vi "VisitSites.vi"(0 "Microsites":T3(array[cluster]), 4 "Path":path, 7 "UiDefinition":T2, 13 "CurrentPositionIndex":i32) -> ()   [LabVIEW 2020]
uses:
  UIReferences.ctl
  C:/Users/User/Desktop/Automation/CurrentVersion/LabviewDXFViewer/bin/Release/LabviewDXFViewer.exe
  LabviewDXFViewer/bin/Release/LabviewDXFViewer.exe
  Control 2.ctl
  <vilib>/Utility/file.llb/Write Delimited Spreadsheet (string).vi
panel:
  out "error out 17":errorcluster
  out "error out 16":errorcluster
  out "error out 15":errorcluster
  out "error out 14":errorcluster
  out "error out 13":errorcluster
  out "error out 12":errorcluster
  out "error out 11":errorcluster
  out "error out 10":errorcluster
  out "error out 9":errorcluster
  out "error out 8":errorcluster
  out "error out 7":errorcluster
  out "error out 6":errorcluster
  out "error out 5":errorcluster
  out "error out 4":errorcluster
  out "IV Curves":T1
  out "error out 3":errorcluster
  out "error out 2":errorcluster
  out "error out":errorcluster
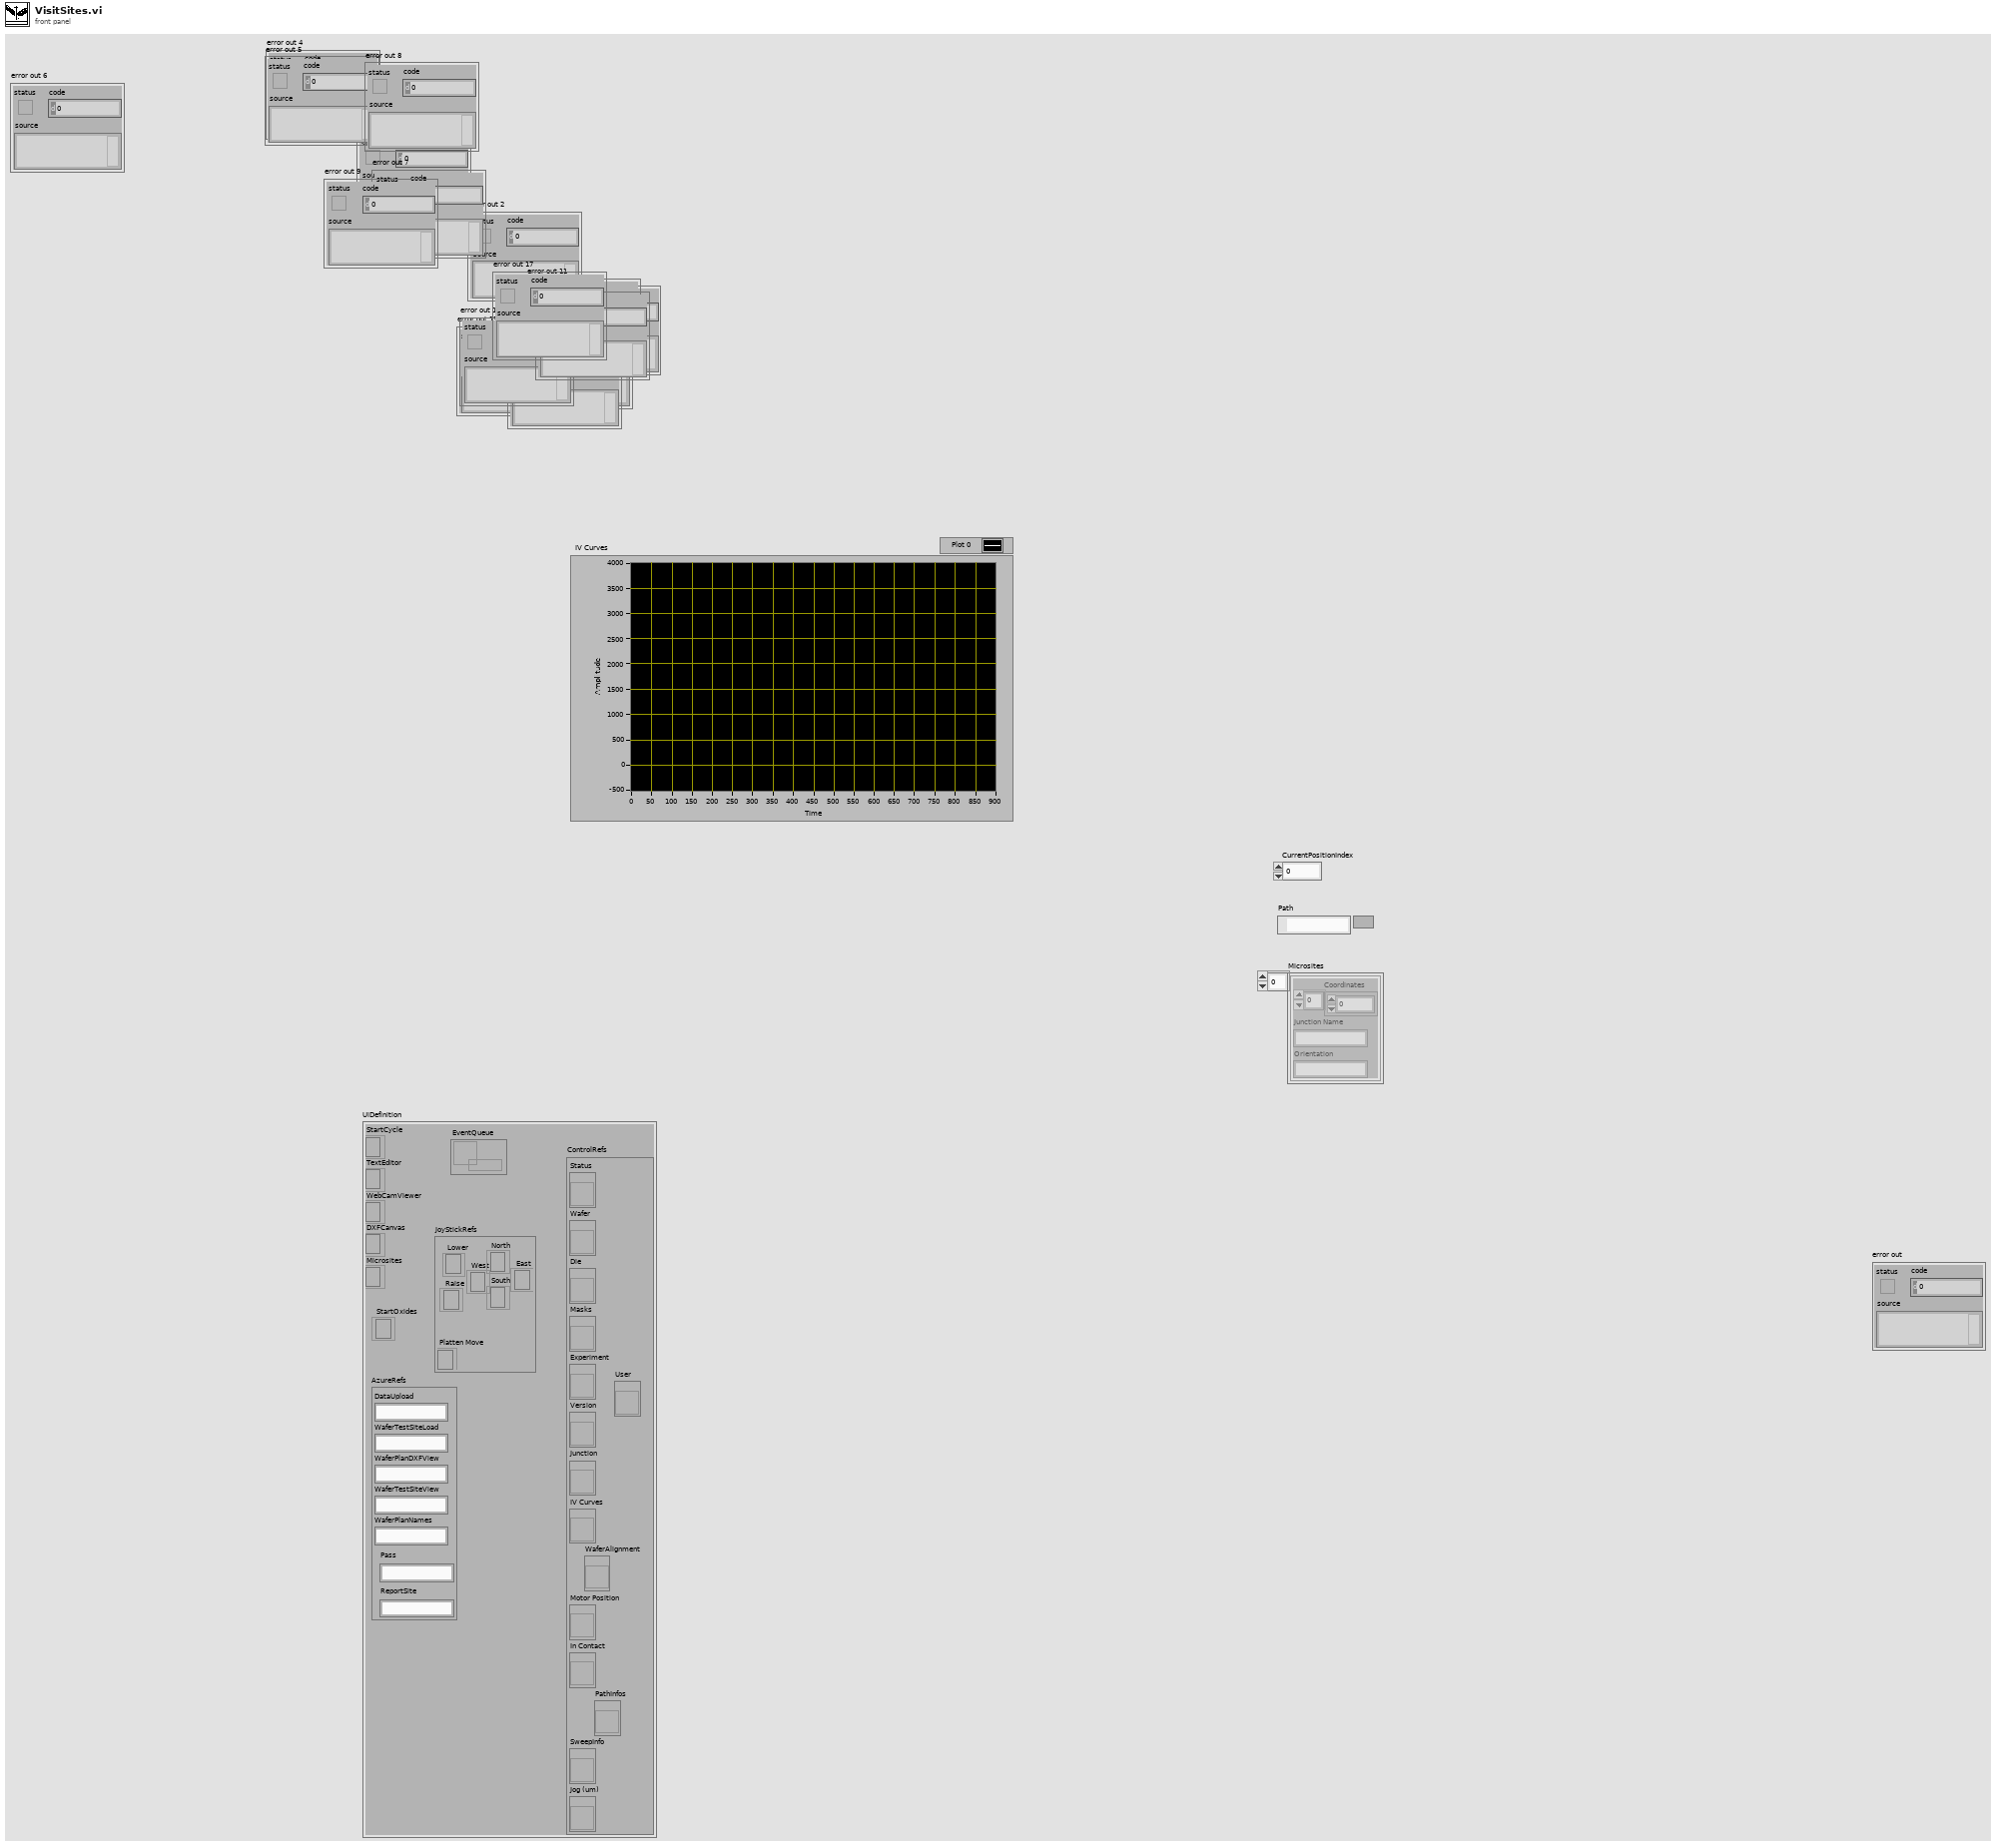
[diagram p1: front panel]
types:
  T1 = typedef "Control 2.ctl" = cluster{"Y":dbl[], "Current (A)":dbl[]}
  T2 = typedef "UIReferences.ctl" = cluster{"StartCycle":refnum<k24>, "TextEditor":refnum<k24>, "WebCamViewer":refnum<k24>, "DXFCanvas":refnum<k24>, "Microsites":refnum<k24>, "JoyStickRefs":cluster{"North":refnum<k24>, "Lower":refnum<k24>, "Raise":refnum<k24>, "Platten Move":refnum<k24>, "West":refnum<k24>, "East":refnum<k24>, "South":refnum<k24>}, "AzureRefs":cluster{"DataUpload":string, "WaferTestSiteLoad":string, "WaferPlanDXFView":string, "WaferTestSiteView":string, "WaferPlanNames":string, "Pass":string, "ReportSite":string}, "ControlRefs":cluster{"Status":refnum<vi>, "Wafer":refnum<vi>, "Die":refnum<vi>, "Masks":refnum<vi>, "Experiment":refnum<vi>, "Version":refnum<vi>, "Junction":refnum<vi>, "IV Curves":refnum<vi>, "Motor Position":refnum<vi>, "In Contact":refnum<vi>, "SweepInfo":refnum<vi>, "Jog (um)":refnum<vi>, "PathInfos":refnum<vi>, "User":refnum<vi>, "WaferAlignment":refnum<vi>}, "EventQueue":refnum<queue>, "StartOxides":refnum<k24>}
  T3 = cluster{"Coordinates":dbl[], "Junction Name":string, "Orientation":string}[]
  T4 = cluster{"Coordinates":dbl[], "Junction Name":string, "Orientation":string}
  T5 = typedef "WaferAlignmentType.ctl" = cluster{"Wafer Units to microns":dbl, "Rotation Misalign":dbl[], "Scale Misalign":dbl, "Steps Per micron":dbl, "Position 1":i32[], "Position 2":i32[], "Lift Distance":i32, "Position 3":i32[], "Jog Height":i32}
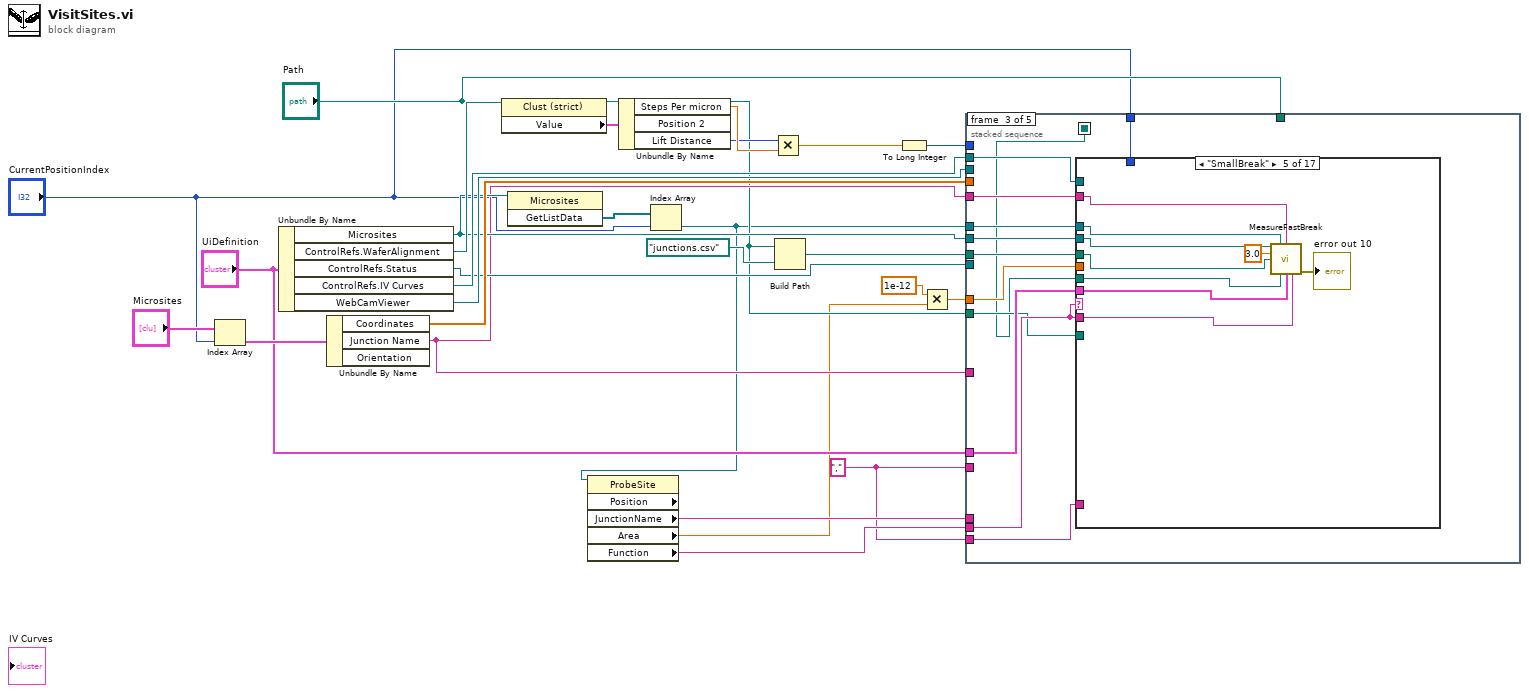
[diagram p0: block diagram]
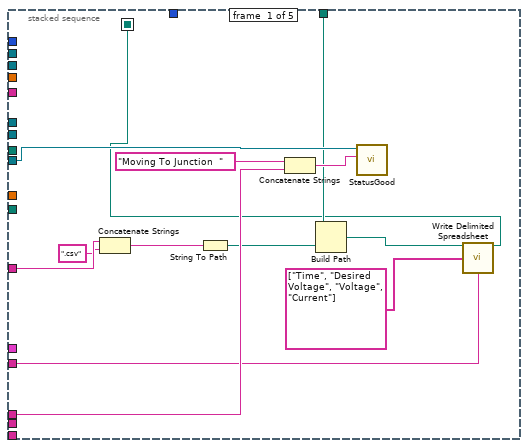
[diagram p2: hidden frame]
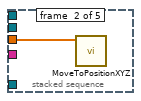
[diagram p3: hidden frame]
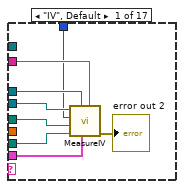
[diagram p4: hidden frame]
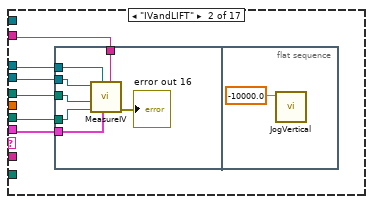
[diagram p5: hidden frame]
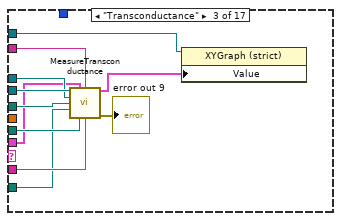
[diagram p6: hidden frame]
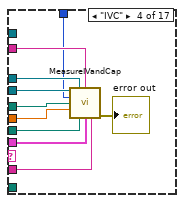
[diagram p7: hidden frame]
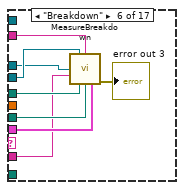
[diagram p8: hidden frame]
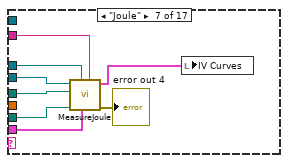
[diagram p9: hidden frame]
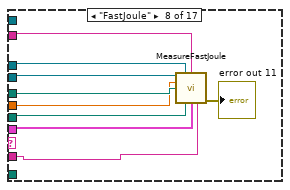
[diagram p10: hidden frame]
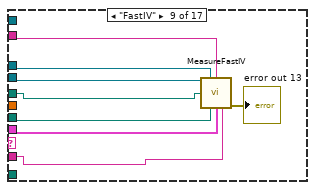
[diagram p11: hidden frame]
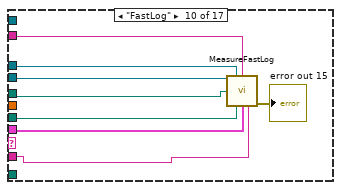
[diagram p12: hidden frame]
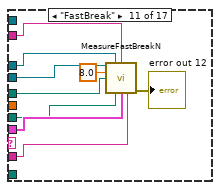
[diagram p13: hidden frame]
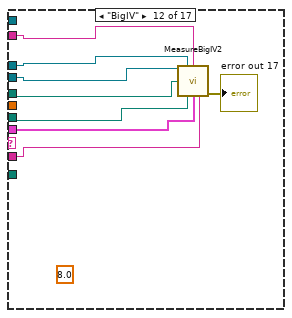
[diagram p14: hidden frame]
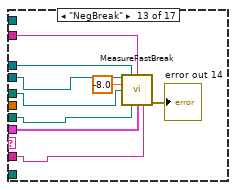
[diagram p15: hidden frame]
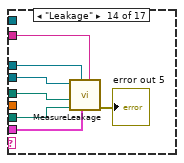
[diagram p16: hidden frame]
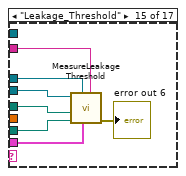
[diagram p17: hidden frame]
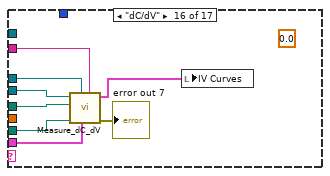
[diagram p18: hidden frame]
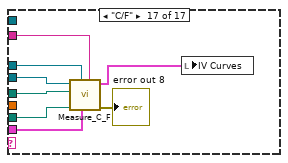
[diagram p19: hidden frame]
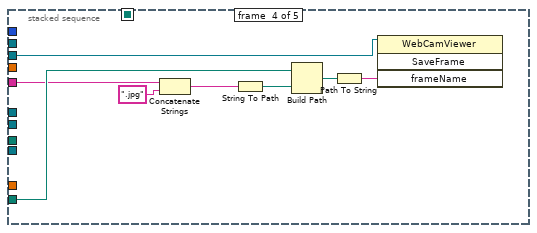
[diagram p20: hidden frame]
diagram:
  w6 = "," ("delimiter (\\t)")
  n1 = Index Array(array="Microsites", index="CurrentPositionIndex") -> (element=w22:T4)
  n2 = Unbundle By Name("UiDefinition") -> ("Microsites"=w9:refnum<k24>, "ControlRefs.WaferAlignment"=w20:refnum<vi>, "ControlRefs.Status"=w7:refnum<vi>, "ControlRefs.IV Curves"=w15:refnum<vi>, "WebCamViewer"=w13:refnum<k24>)
  n3 = Unbundle By Name(w22) -> ("Coordinates"=w25:dbl[], "Junction Name"=w5:string)  [unwired: 1 out]
  n4 = property class="Clust (strict)"(reference=w20) -> ("Value"=w19:T5)  [unwired: 1 in, 2 out]
  n5 = invoke class="Microsites" method="GetListData"(reference=w9) -> ("GetListData"=w21:refnum<k24>[])  [unwired: 2 in, 2 out]
  n6 = Unbundle By Name(w19) -> ("Steps Per micron"=w17:dbl, "Lift Distance"=w16:i32)  [unwired: 1 out]
  n7 = Index Array(array=w21, index="CurrentPositionIndex") -> (element=w2:refnum<k24>)
  n8 = property class="ProbeSite" props=["Position", "JunctionName", "Area", "Function"](reference=w2) -> ("JunctionName"=w8:string, "Area"=w3:dbl, "Function"=w10:string)  [unwired: 1 in, 3 out]
  n9 = Multiply(x=w16, y=w17) -> (x*y=w18:dbl)
  n10 = Build Path(base path="Path", name or relative path=path "junctions.csv") -> (appended path=w26:path)
  n11 = To Long Integer(number=w18) -> (32bit integer=w27:i32)
  n12 = Multiply(x=1e-12, y=w3) -> (x*y=w12:dbl)
  n13 = stacked-sequence {
    seq-local: [w28 _ _ _ _] -> [_ _ w43 _ _]
    tunnel: w27 -> [_ _ _ _ w212]
    tunnel: w26 -> [_ _ w53 _ _]
    tunnel: w25 -> [_ w41 _ _ _]
    tunnel: w5 -> [_ _ w52 w205 _]
    tunnel: w15 -> [_ _ w45 _ _]
    tunnel: "UiDefinition" -> [_ _ w50 _ _]
    tunnel: w6 -> [_ _ w51 _ _]
    tunnel: w13 -> [_ _ _ w210 _]
    tunnel: "Path" -> [_ _ w44 w209 _]
    tunnel: w12 -> [_ _ w49 _ _]
    tunnel: w10 -> [_ _ w46 _ _]
    tunnel: w9 -> [_ _ w48 _ _]
    tunnel: w2 -> [_ _ w47 _ _]
    tunnel: w8 -> [w38 _ _ _ _]
    tunnel: w7 -> [w37 _ _ _ _]
    tunnel: w6 -> [w32 _ _ _ _]
    tunnel: w5 -> [w31 _ _ _ _]
    tunnel: "Path" -> [w29 _ _ _ _]
    tunnel: "CurrentPositionIndex" -> [_ _ w42 _ _]
    frame #0 {
      n14 = Concatenate Strings(w31, ".csv" ("string")) -> (w34:string)
      n15 = String To Path(string=w34) -> (path=w35:path)
      n16 = Concatenate Strings("Moving To Junction  " ("Text.Text"), w38) -> (w40:string)
      n17 = Build Path(base path=w29, name or relative path=w35) -> (appended path=w36:path)
      n18 = call "StatusGood.vi"("Text.Text"=w40, "String in"=w37) -> ()  [unwired: 10 in]
      n19 = call-poly <vilib>:"Write Delimited Spreadsheet.vi"("file path (dialog if empty)"=w36, "1D data"=string[] ["Time", "Desired Voltage", "Voltage", "Current"], "delimiter (\\t)"=w32) -> ("new file path (Not A Path if cancelled)"=w28:path)  [unwired: 11 in, 1 out]
    }
    frame #1 {
      n20 = call "MoveToPositionXYZ.vi"("Array"=w41) -> ()  [unwired: 11 in]
    }
    frame #2 {
      n21 = case shown="\"SmallBreak\"" w46 {
        tunnel: w53 -> [w59 w64 w82 w96 w97 w113 w116 w124 w134 w142 w147 w159 w165 w176 w182 w191 w199]
        tunnel: w52 -> [w58 w67 w76 w95 w104 w107 w117 w129 w137 w145 w154 w158 w170 w175 w183 w190 w198]
        tunnel: w43 -> [w60 w63 w83 w94 w99 w112 w118 w123 w133 w141 w149 w160 w164 w174 w181 w189 w196]
        tunnel: w51 -> [_ _ _ _ _ _ _ _ _ _ _ _ _ _ _ _ _]
        tunnel: w50 -> [w57 w62 w80 w93 w100 w109 w115 w125 w132 w140 w150 w161 w167 w173 w180 w188 w197]
        tunnel: w49 -> [_ _ _ w92 _ _ _ w122 _ _ _ _ _ _ _ _ _]
        tunnel: w48 -> [w56 w65 w85 w91 w102 w111 w120 w127 w135 w143 w152 w156 w166 w177 w184 w192 w200]
        tunnel: w47 -> [w55 w66 w84 w90 w103 w110 w119 w128 w136 w144 w153 w157 w169 w178 w185 w193 w201]
        tunnel: w46 -> [_ _ w81 w89 w101 w108 _ w126 w131 w139 w151 w162 w168 _ _ _ _]
        tunnel: w45 -> [_ _ w79 _ _ _ _ _ _ _ _ _ _ _ _ _ _]
        tunnel: w44 -> [_ _ w77 _ _ _ _ _ _ _ _ _ _ _ _ _ _]
        tunnel: w42 -> [w54 _ _ w87 _ _ _ _ _ _ _ _ _ _ _ _ _]
        frame "IV", Default {
          n22 = call "MeasureIV.vi"("Junction Name"=w58, "UiDefinition"=w57, ".NET Refnum"=w55, "new file path (Not A Path if cancelled)"=w60, "appended path"=w59, "CurrentPositionIndex"=w54, ".NET Refnum in"=w56) -> ("error out"=→"error out 2":errorcluster)  [unwired: 4 in]
        }
        frame "IVandLIFT" {
          n23 = flat-sequence {
            tunnel: w67 -> [w73]
            tunnel: w66 -> [w72]
            tunnel: w65 -> [w71]
            tunnel: w64 -> [w70]
            tunnel: w63 -> [w69]
            tunnel: w62 -> [w68]
            frame #0 {
              n24 = call "MeasureIV.vi"("Junction Name"=w73, "UiDefinition"=w68, ".NET Refnum"=w72, "new file path (Not A Path if cancelled)"=w69, "appended path"=w70, ".NET Refnum in"=w71) -> ("error out"=→"error out 16":errorcluster)  [unwired: 5 in]
            }
            frame #1 {
              n25 = call "JogVertical.vi"("Numeric"=-10000.0) -> ()  [unwired: 11 in]
            }
          }
        }
        frame "Transconductance" {
          n26 = call "MeasureTransconductance.vi"(".NET Refnum in"=w85, "UiDefinition"=w80, "Junction Name"=w76, ".NET Refnum"=w84, "appended path"=w82, "Path"=w77, "new file path (Not A Path if cancelled)"=w83, "Function"=w81) -> ("Cluster"=w78:cluster{dbl[], dbl[]}, "error out"=→"error out 9":errorcluster)  [unwired: 6 in]
          n27 = property class="XYGraph (strict)"(reference=w79, "Value"=w78) -> ()  [unwired: 1 in, 2 out]
        }
        frame "IVC" {
          n28 = call "MeasureIVandCap.vi"(".NET Refnum in"=w91, ".NET Refnum"=w90, "Junction Name"=w95, "CurrentPositionIndex"=w87, "appended path"=w96, "Numeric"=w92, "new file path (Not A Path if cancelled)"=w94, "UiDefinition"=w93, "Function"=w89) -> ("error out"=→"error out":errorcluster)  [unwired: 6 in]
        }
        frame "SmallBreak" {
          n29 = call "MeasureFastBreak.vi"(".NET Refnum in"=w102, ".NET Refnum"=w103, "Junction Name"=w104, "Maxiumum Voltage"=3.0, "appended path"=w97, "new file path (Not A Path if cancelled)"=w99, "UiDefinition"=w100, "Function"=w101) -> ("error out"=→"error out 10":errorcluster)  [unwired: 7 in]
        }
        frame "Breakdown" {
          n30 = call "MeasureBreakdown.vi"("Microsites"=w111, "Junction Name"=w107, ".NET Refnum"=w110, "Function"=w108, "appended path"=w113, "new file path (Not A Path if cancelled)"=w112, "UiDefinition"=w109) -> ("error out"=→"error out 3":errorcluster)  [unwired: 8 in]
        }
        frame "Joule" {
          n31 = call "MeasureJoule.vi"("Junction Name"=w117, "UiDefinition"=w115, ".NET Refnum"=w119, "new file path (Not A Path if cancelled)"=w118, "appended path"=w116, ".NET Refnum in"=w120) -> ("error out"=→"error out 4":errorcluster, "Cluster"=w114:cluster{dbl[], dbl[]})  [unwired: 4 in]
          n32 = local write "IV Curves"(w114) -> ()
        }
        frame "FastJoule" {
          n33 = call "MeasureFastJoule.vi"(".NET Refnum in"=w127, ".NET Refnum"=w128, "Junction Name"=w129, "Maxiumum Voltage"=w122, "appended path"=w124, "new file path (Not A Path if cancelled)"=w123, "UiDefinition"=w125, "Function"=w126) -> ("error out"=→"error out 11":errorcluster)  [unwired: 7 in]
        }
        frame "FastIV" {
          n34 = call "MeasureFastIV.vi"(".NET Refnum in"=w135, ".NET Refnum"=w136, "Junction Name"=w137, "appended path"=w134, "new file path (Not A Path if cancelled)"=w133, "UiDefinition"=w132, "Function"=w131) -> ("error out"=→"error out 13":errorcluster)  [unwired: 8 in]
        }
        frame "FastLog" {
          n35 = call "MeasureFastLog.vi"(".NET Refnum in"=w143, ".NET Refnum"=w144, "Junction Name"=w145, "appended path"=w142, "new file path (Not A Path if cancelled)"=w141, "UiDefinition"=w140, "Function"=w139) -> ("error out"=→"error out 15":errorcluster)  [unwired: 8 in]
        }
        frame "FastBreak" {
          n36 = call "MeasureFastBreakN.vi"(".NET Refnum in"=w152, ".NET Refnum"=w153, "Junction Name"=w154, "MaxVoltage"=8.0 ("Maxiumum Voltage"), "appended path"=w147, "new file path (Not A Path if cancelled)"=w149, "UiDefinition"=w150, "Function"=w151) -> ("error out"=→"error out 12":errorcluster)  [unwired: 7 in]
        }
        frame "BigIV" {
          (unwired) 8.0 ("Maxiumum Voltage")
          n37 = call "MeasureBigIV2.vi"(".NET Refnum in"=w156, ".NET Refnum"=w157, "Junction Name"=w158, "appended path"=w159, "new file path (Not A Path if cancelled)"=w160, "UiDefinition"=w161, "Function"=w162) -> ("error out"=→"error out 17":errorcluster)  [unwired: 8 in]
        }
        frame "NegBreak" {
          n38 = call "MeasureFastBreak.vi"(".NET Refnum in"=w166, ".NET Refnum"=w169, "Junction Name"=w170, "Maxiumum Voltage"=-8.0, "appended path"=w165, "new file path (Not A Path if cancelled)"=w164, "UiDefinition"=w167, "Function"=w168) -> ("error out"=→"error out 14":errorcluster)  [unwired: 7 in]
        }
        frame "Leakage" {
          n39 = call "MeasureLeakage.vi"("Junction Name"=w175, "UiDefinition"=w173, ".NET Refnum"=w178, "new file path (Not A Path if cancelled)"=w174, "appended path"=w176, ".NET Refnum in"=w177) -> ("error out"=→"error out 5":errorcluster)  [unwired: 5 in]
        }
        frame "Leakage_Threshold" {
          n40 = call "MeasureLeakageThreshold.vi"("Junction Name"=w183, "UiDefinition"=w180, ".NET Refnum"=w185, "new file path (Not A Path if cancelled)"=w181, "appended path"=w182, ".NET Refnum in"=w184) -> ("error out"=→"error out 6":errorcluster)  [unwired: 5 in]
        }
        frame "dC/dV" {
          (unwired) 0.0 ("Vpp")
          n41 = call "Measure_dC_dV.vi"("Junction Name"=w190, "UiDefinition"=w188, ".NET Refnum"=w193, "new file path (Not A Path if cancelled)"=w189, "appended path"=w191, ".NET Refnum in"=w192) -> ("error out"=→"error out 7":errorcluster, "Cluster"=w187:cluster{dbl[], dbl[]})  [unwired: 4 in]
          n42 = local write "IV Curves"(w187) -> ()
        }
        frame "C/F" {
          n43 = call "Measure_C_F.vi"("Junction Name"=w198, "UiDefinition"=w197, ".NET Refnum"=w201, "new file path (Not A Path if cancelled)"=w196, "appended path"=w199, ".NET Refnum in"=w200) -> ("error out"=→"error out 8":errorcluster, "Cluster"=w195:cluster{dbl[], dbl[]})  [unwired: 4 in]
          n44 = local write "IV Curves"(w195) -> ()
        }
      }
    }
    frame #3 {
      n45 = Concatenate Strings(w205, ".jpg" ("string")) -> (w208:string)
      n46 = String To Path(string=w208) -> (path=w206:path)
      n47 = Build Path(base path=w209, name or relative path=w206) -> (appended path=w204:path)
      n48 = Path To String(path=w204) -> (string=w203:string)
      n49 = invoke class="WebCamViewer" method="SaveFrame"(reference=w210, "frameName"=w203) -> ()  [unwired: 2 in, 4 out]
    }
    frame #4 {
      # "Move Up"
      n50 = Negate(x=w212) -> (-x=w211:i32)
      n51 = call "JogVertical.vi"("Numeric"=w211) -> ()  [unwired: 11 in]
    }
  }
